vi "Stepping Motor v1.2.vi"() -> ()   [LabVIEW 2012]
uses:
  <vilib>/DAQmx/write.llb/DAQmx Write (Digital U8 1Chan 1Samp).vi
  <vilib>/DAQmx/create/channels.llb/DAQmx Create Channel (DO-Digital Output).vi
  <vilib>/DAQmx/miscellaneous.llb/DAQmx Fill In Error Info.vi
panel:
  in  "lines":tag
  out "Array":bool[](array[boolean])
  out "Data to Write":u32=255 format="%x"
  in  "stop":bool
  in  "Array 2":bool[][](array[boolean])=[[TRUE, FALSE, FALSE, TRUE], [TRUE, TRUE, FALSE, FALSE], [FALSE, TRUE, TRUE, FALSE], [FALSE, FALSE, TRUE, TRUE]]
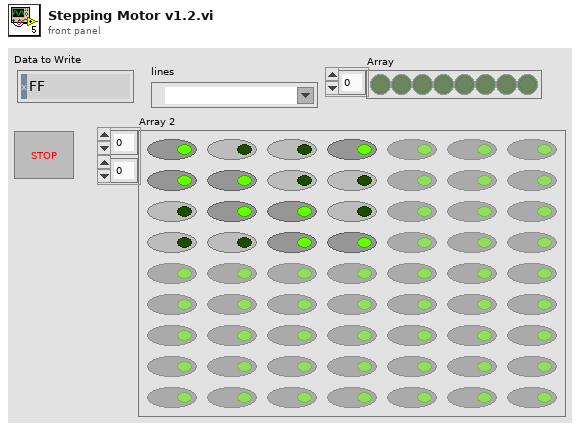
[diagram p1: front panel]
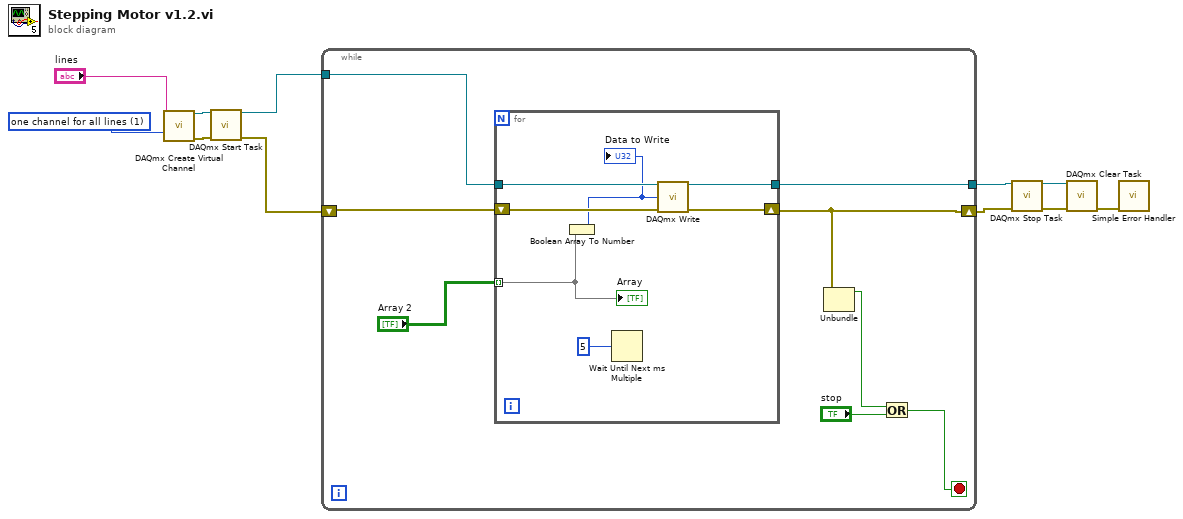
[diagram p0: block diagram]
diagram:
  w5 = 1 items=["one channel for each line", "one channel for all lines"] ("line grouping")
  n1 = call-poly <vilib>:"DAQmx Create Virtual Channel.vi"("lines"="lines", "line grouping"=w5) -> ("task out"=w4:refnum<k21>, "error out"=w3:errorcluster)  [unwired: 12 in]
  n2 = call <vilib>:"DAQmx Start Task.vi"("task/channels in"=w4, "error in"=w3) -> ("task out"=w2:refnum<k21>, "error out"=w1:errorcluster)  [unwired: 12 in]
  n3 = while {
    shift-right: [w17] -> w7
    shift-left: w1 -> [w13]
    tunnel: [w18] -> w8
    tunnel: w2 -> [w12]
    stop <- w14 stop-if-true
    n4 = for {
      tunnel: w12 -> [w25]
      tunnel: [w24] -> w18
      tunnel: "Array 2" -> [w20] mode=indexing
      shift-right: [w22] -> w17
      shift-left: w13 -> [w26]
      n5 = Boolean Array To Number(Boolean array=w20) -> (number=w21:u32)
      "Data to Write" <- w21
      n6 = Wait Until Next ms Multiple(millisecond multiple=5) -> ()  [unwired: 1 out]
      n7 = call-poly <vilib>:"DAQmx Write.vi"("task/channels in"=w25, "data"=w21, "error in"=w26) -> ("task out"=w24:refnum<k21>, "error out"=w22:errorcluster)  [unwired: 10 in, 1 out]
      "Array" <- w20
    }
    n8 = Unbundle(w17) -> ("status"=w16:bool)  [unwired: 2 out]
    n9 = Or(x=w16, y="stop") -> (x .or. y?=w14:bool)
  }
  n10 = call <vilib>:"DAQmx Stop Task.vi"("task/channels in"=w8, "error in"=w7) -> ("task out"=w10:refnum<k21>, "error out"=w9:errorcluster)  [unwired: 12 in]
  n11 = call <vilib>:"DAQmx Clear Task.vi"("task in"=w10, "error in"=w9) -> ("error out"=w11:errorcluster)  [unwired: 13 in]
  n12 = call <vilib>:"Simple Error Handler.vi"("error in (no error)"=w11) -> ()  [unwired: 4 in, 5 out]
